vi "StartTest_AfterStartTestSuite_AddsNestedTestCase.vi"() -> ()   [LabVIEW 2017, in "ResultTreeListenerTest.lvlib"]
uses:
  ResultTreeListenerTest.lvlib
  ResultTreeListener/ResultTreeListener.lvclass
  ResultTree/ResultTree.lvclass
  b9be8222-4629-4de4-b646-ac532e0c1106.vi
  Support/FakeTestCase/FakeTestCase.lvclass
  Support/FakeTestSuite/FakeTestSuite.lvclass
  C:/Users/de200256/Code/neuperger/lvunit/TestSuite/TestSuite.lvclass
  C:/Users/de200256/Code/neuperger/lvunit/Test/Test.lvclass
panel:
  out "error out":errorcluster
  in  "Tree":string(tree)
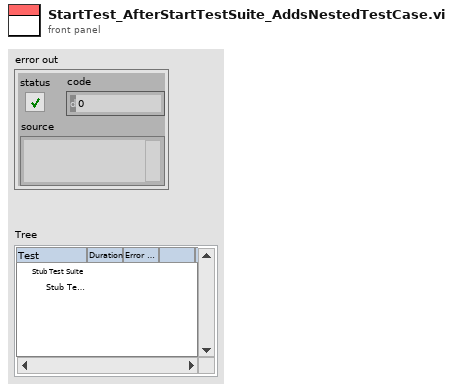
[diagram p1: front panel]
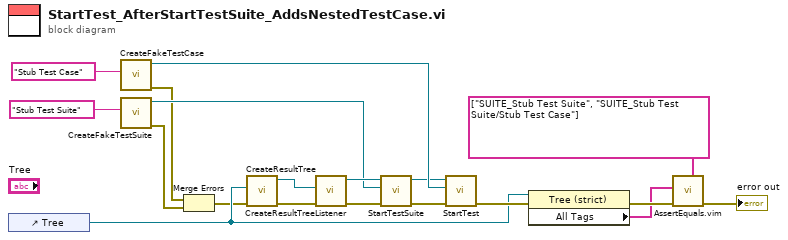
[diagram p0: block diagram]
diagram:
  n1 = control-ref of="Tree"() -> (w12:refnum<vi>)
  n2 = call "CreateFakeTestCase.vi"("Name"="Stub Test Case") -> ("error out"=w2:errorcluster, "FakeTestCase out"=w15:refnum<class "FakeTestCase.lvclass">)  [unwired: 9 in]
  n3 = call "CreateFakeTestSuite.vi"("Name"="Stub Test Suite") -> ("error out"=w1:errorcluster, "FakeTestSuite out"=w4:refnum<class "FakeTestSuite.lvclass">)  [unwired: 9 in]
  n4 = Merge Errors(w2, w1) -> (w3:errorcluster)
  n5 = call "CreateResultTree.vi"("error in (no error)"=w3, "Tree Refnum"=w12) -> ("error out"=w19:errorcluster, "ResultTree out"=w18:refnum<class "ResultTree.lvclass">)  [unwired: 8 in]
  n6 = call "CreateResultTreeListener.vi"("error in (no error)"=w19, "ResultTree"=w18) -> ("error out"=w6:errorcluster, "ResultTreeListener out"=w8:refnum<class "ResultTreeListener.lvclass">)  [unwired: 8 in]
  n7 = call-dynamic "StartTestSuite.vi"("error in (no error)"=w6, "TestSuite"=w4, "ResultTreeListener in"=w8) -> ("error out"=w5:errorcluster, "ResultTreeListener out"=w7:refnum<class "ResultTreeListener.lvclass">)  [unwired: 7 in]
  n8 = call-dynamic "StartTest.vi"("error in (no error)"=w5, "Test"=w15, "ResultTreeListener in"=w7) -> ("error out"=w16:errorcluster)  [unwired: 7 in, 1 out]
  n9 = property class="Tree (strict)"(reference=w12, error in=w16) -> (error out=w13:errorcluster, "All Tags"=w11:string[])  [unwired: 1 out]
  n10 = call "AssertEquals.vim"("Expected"=string[] ["SUITE_Stub Test Suite", "SUITE_Stub Test Suite/Stub Test Case"] ("All Tags"), "error in (no error)"=w13, "Actual"=w11) -> ("error out"=→"error out":errorcluster)  [unwired: 8 in]
